vi "Drive Metric to Loggable.vi"(11 "Drive Metrics":T1) -> (3 "resulting string":string)   [LabVIEW 2015]
uses:
  Drive Metrics.ctl
  Drive States.ctl
  Copilot States.ctl
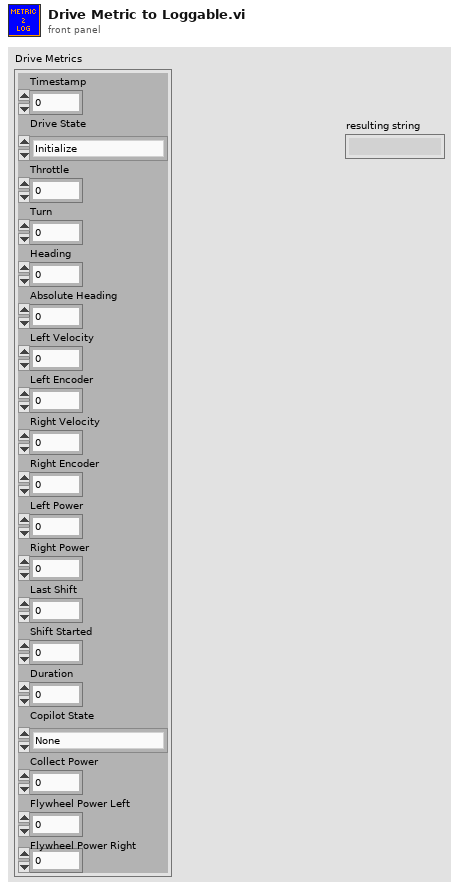
[diagram p1: front panel]
types:
  T1 = typedef "Drive Metrics.ctl" = cluster{"Timestamp":u32, "Drive State":T2, "Throttle":dbl, "Turn":dbl, "Heading":dbl, "Absolute Heading":dbl, "Left Velocity":dbl, "Left Encoder":dbl, "Right Velocity":dbl, "Right Encoder":dbl, "Left Power":dbl, "Right Power":dbl, "Last Shift":u32, "Shift Started":u32, "Duration":i64, "Copilot State":T3, "Collect Power":dbl, "Flywheel Power Left":dbl, "Flywheel Power Right":dbl}
  T2 = typedef "Drive States.ctl" = enum16{"Initialize", "Low Gear", "Up Shift Begin", "Up Shifting", "Up Shift Delay", "High Gear", "Down Shift Begin", "Down Shifting", "Down Shift Delay"}
  T3 = typedef "Copilot States.ctl" = enum16{"None", "Collect", "Eject"}
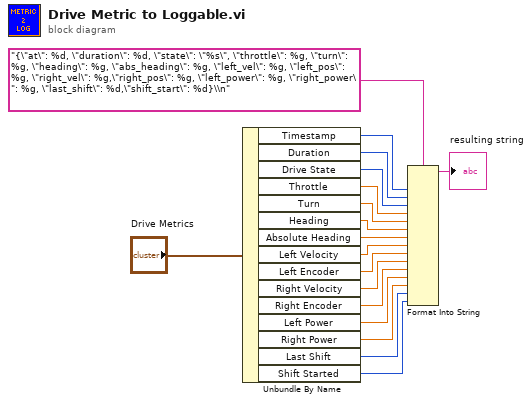
[diagram p0: block diagram]
diagram:
  n1 = Unbundle By Name("Drive Metrics") -> ("Timestamp"=w16:u32, "Duration"=w1:i64, "Drive State"=w2:T2, "Throttle"=w15:dbl, "Turn"=w14:dbl, "Heading"=w13:dbl, "Absolute Heading"=w12:dbl, "Left Velocity"=w11:dbl, "Left Encoder"=w10:dbl, "Right Velocity"=w9:dbl, "Right Encoder"=w8:dbl, "Left Power"=w7:dbl, "Right Power"=w6:dbl, "Last Shift"=w5:u32, "Shift Started"=w4:u32)
  n2 = Format Into String(format string="{\"at\": %d, \"duration\": %d, \"state\": \"%s\", \"throttle\": %g, \"turn\": %g, \"heading\": %g, \"abs_heading\": %g, \"left_vel\": %g, \"left_pos\": %g, \"right_vel\": %g,\"right_pos\": %g, \"left_power\": %g, \"right_power\": %g, \"last_shift\": %d,\"shift_start\": %d}\\n", w16, w1, w2, w15, w14, w13, w12, w11, w10, w9, w8, w7, w6, w5, w4) -> (resulting string=→"resulting string":string)  [unwired: 2 in, 1 out]
